vi "AC_Source_VISA.vi"(3 "error_in":errorcluster, 4 "Parameter":T1, 5 "Mode":T2(ring)=enum."TurnOn", 6 "VISA_in":refnum<visa-resource-name>) -> (0 "error_out":errorcluster, 1 "read buffer":string, 2 "VISA_out":refnum<visa-resource-name>)   [LabVIEW 2019]
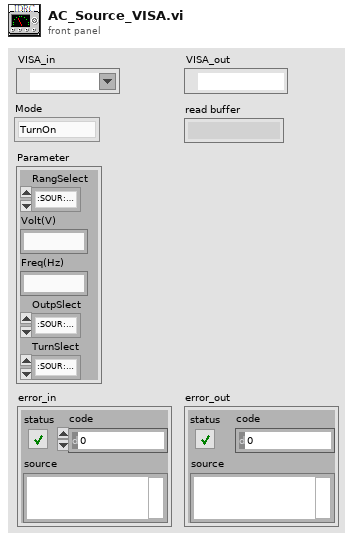
[diagram p1: front panel]
types:
  T1 = cluster{"RangSelect":enum16{":SOUR:RANG LOW;", ":SOUR:RANG HIGH;", ":SOUR:RANG AUTO;"}, "Volt(V)":string, "Freq(Hz)":string, "OutpSlect":enum16{":SOUR:TURN OFF;", ":SOUR:TURN ON;"}, "TurnSlect":enum16{":SOUR:TURN OFF;", ":SOUR:TURN ON;"}}
  T2 = enum16{"SetRange", "SetVoltage", "SetFreq", "OUTP", "TurnOn"}
  T3 = enum16{":SOUR:RANG LOW;", ":SOUR:RANG HIGH;", ":SOUR:RANG AUTO;"}
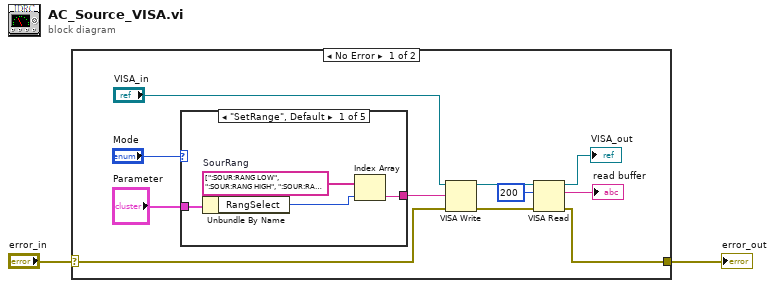
[diagram p0: block diagram]
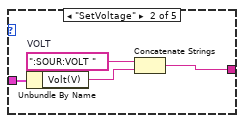
[diagram p2: hidden frame]
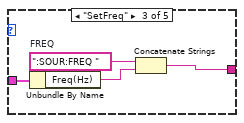
[diagram p3: hidden frame]
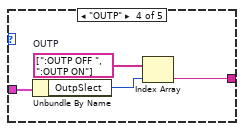
[diagram p4: hidden frame]
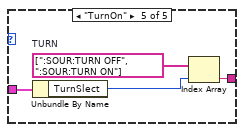
[diagram p5: hidden frame]
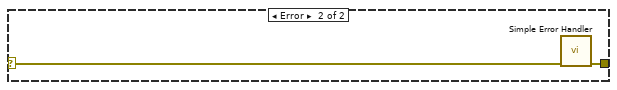
[diagram p6: hidden frame]
diagram:
  n1 = case shown="No Error" "error_in" {
    selector: "error_in" -> [w10 w35]
    tunnel: [w7 w34] -> w1
    frame No Error {
      n2 = case shown="\"SetRange\", Default" "Mode" {
        tunnel: "Parameter" -> [w16 w20 w24 w28 w32]
        tunnel: [w14 w18 w22 w27 w30] -> w11
        frame "SetRange", Default {
          w17 = string[] [":SOUR:RANG LOW", ":SOUR:RANG HIGH", ":SOUR:RANG AUTO;"]  # SourRang
          n3 = Unbundle By Name(w16) -> ("RangSelect"=w15:T3)
          n4 = Index Array(array=w17, index=w15) -> (element=w14:string)
        }
        frame "SetVoltage" {
          w21 = ":SOUR:VOLT "  # VOLT
          n5 = Unbundle By Name(w20) -> ("Volt(V)"=w19:string)
          n6 = Concatenate Strings(w21, w19) -> (w18:string)
        }
        frame "SetFreq" {
          w25 = ":SOUR:FREQ "  # FREQ
          n7 = Unbundle By Name(w24) -> ("Freq(Hz)"=w23:string)
          n8 = Concatenate Strings(w25, w23) -> (w22:string)
        }
        frame "OUTP" {
          w29 = string[] [":OUTP OFF ", ":OUTP ON"]  # OUTP
          n9 = Unbundle By Name(w28) -> ("OutpSlect"=w26:enum16{":SOUR:TURN OFF;", ":SOUR:TURN ON;"})
          n10 = Index Array(array=w29, index=w26) -> (element=w27:string)
        }
        frame "TurnOn" {
          w33 = string[] [":SOUR:TURN OFF", ":SOUR:TURN ON"]  # TURN
          n11 = Unbundle By Name(w32) -> ("TurnSlect"=w31:enum16{":SOUR:TURN OFF;", ":SOUR:TURN ON;"})
          n12 = Index Array(array=w33, index=w31) -> (element=w30:string)
        }
      }
      n13 = VISA Write(VISA resource name="VISA_in", write buffer=w11, error in (no error)=w10) -> (VISA resource name out=w6:refnum<visa-resource-name>, error out=w8:errorcluster)  [unwired: 1 out]
      n14 = VISA Read(VISA resource name=w6, byte count=u32 200, error in (no error)=w8) -> (VISA resource name out=→"VISA_out":refnum<visa-resource-name>, read buffer=→"read buffer":string, error out=w7:errorcluster)  [unwired: 1 out]
    }
    frame Error {
      n15 = call <vilib>:"Simple Error Handler.vi"("error in (no error)"=w35) -> ("error out"=w34:errorcluster)  [unwired: 4 in, 4 out]
    }
  }
  "error_out" <- w1
